vi "Actor Core.vi"(8 "error in":errorcluster, 11 "UI Main Startup in":refnum<class "UI Main Startup.lvclass">) -> (0 "error out":errorcluster, 3 "Actor out":refnum<class "Actor.lvclass">)   [LabVIEW 2020, in "UI Main Startup.lvlib" / "UI Main Startup.lvclass"]
doc: "(<B>Filename</B>: Actor Framework.lvlib:Actor.lvclass:Actor Core.vi)\n\nReceives messages to the actor, reacts to them, and initiates any error handling that may shut the actor down.\n\nDescendant classes may override this VI to append parallel tasks for the actor to complete while it handles messages. Overrides use the Call Parent Class Method node."
uses:
  UI Main Startup.lvclass
  C:/Program Files (x86)/National Instruments/LabVIEW 2020/vi.lib/ActorFramework/Actor/Actor.lvclass
  <vilib>/ActorFramework/Actor/Actor.lvclass
  <vilib>/ActorFramework/Actor/Actor.lvclass/Actor.ctl
  UI Main/UI Main Messages/Update Sub Panel Msg/Update Sub Panel Msg.lvclass/Update Sub Panel Msg.ctl
  <vilib>/ActorFramework/Message Enqueuer/Message Enqueuer.lvclass/Message Enqueuer.ctl
  <vilib>/ActorFramework/Message Enqueuer/Enqueue.vi
  UI Main/UI Main Messages/Update Sub Panel Msg/Update Sub Panel Msg.lvclass
  C:/Program Files (x86)/National Instruments/LabVIEW 2020/vi.lib/ActorFramework/Message/Message.lvclass
  <vilib>/ActorFramework/Message Priority Queue/Priority Enqueue.vi
panel:
  in  "String":string
  in  "Cancel Button":bool
  in  "OK Button":bool
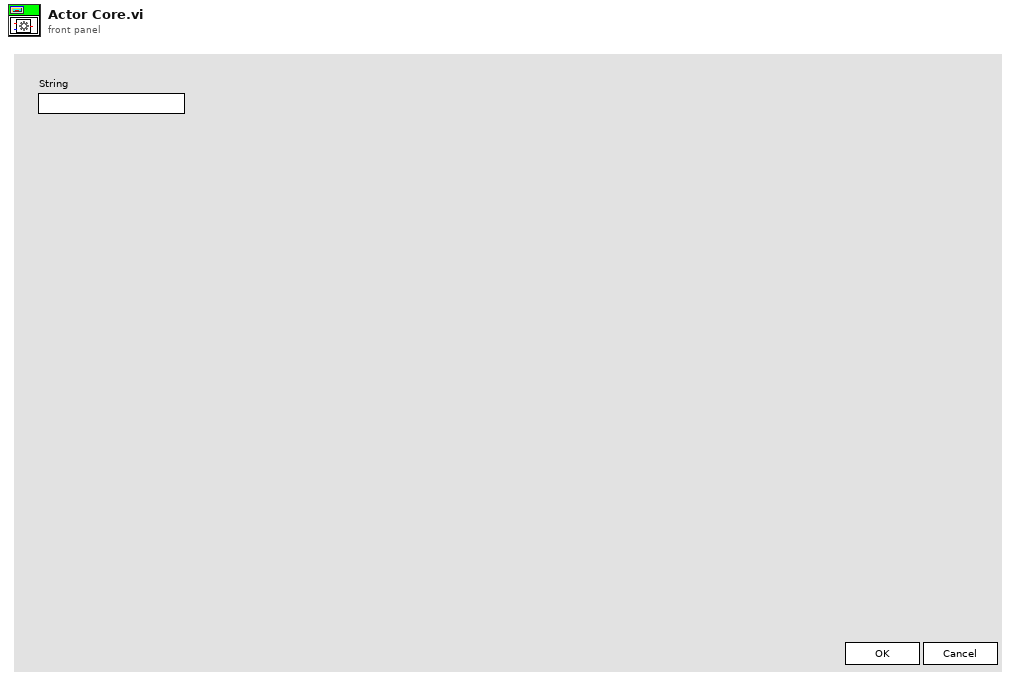
[diagram p1: front panel]
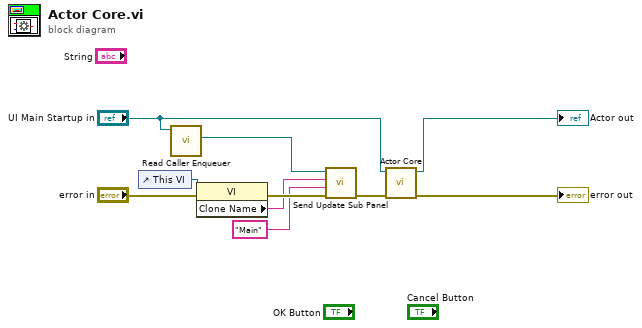
[diagram p0: block diagram]
diagram:
  n1 = control-ref of="This VI"() -> (w7:refnum<vi>)
  n2 = call <vilib>:"Read Caller Enqueuer.vi"("Actor"="UI Main Startup in") -> ("Caller Enqueuer"=w3:refnum<class "Message Enqueuer.lvclass">)  [unwired: 10 in]
  n3 = property class="VI"(reference=w7, error in="error in") -> (error out=w5:errorcluster, "Clone Name"=w2:string)  [unwired: 1 out]
  n4 = call "Send Update Sub Panel.vi"("error in (no error)"=w5, "UI Section"="Main", "Clone Name"=w2, "Message Enqueuer"=w3) -> ("error out"=w4:errorcluster)  [unwired: 6 in, 1 out]
  n5 = call-parent "Actor Core.vi"("error in"=w4, "Actor in"="UI Main Startup in") -> ("error out"=→"error out":errorcluster, "Actor out"=→"Actor out":refnum<class "Actor.lvclass">)  [unwired: 8 in]
